vi "Main UI.vi"(8 "error in (no error)":errorcluster, 11 "picoG in":refnum<class "picoG.lvclass">) -> (0 "error out":errorcluster, 3 "picoG out":refnum<class "picoG.lvclass">)   [LabVIEW 2020, in "PicoG-App.lvlib" / "picoG.lvclass"]
uses:
  picoG.lvclass
  UI State.ctl
  picoG.lvclass/picoG.ctl
  AppListPanel/AppListPanel.lvclass
  C:/Program Files (x86)/National Instruments/LabVIEW 2020/vi.lib/IlluminatedG/IG OOPanel/OOPanel/Panel/Panel.lvclass
  DeviceListPanel/DeviceListPanel.lvclass
  GettingStarted/GettingStarted.lvclass
  PlatformListPanel/PlatformListPanel.lvclass
  AppDetailPanel/AppDetailPanel.lvclass
  DeviceDetailPanel/DeviceDetailPanel.lvclass
  PlatformConfigPanel/PlatformConfigPanel.lvclass
  AppListPanel/Panel.vi
  ViaApp/ViaApp.lvclass
  Builds/picoG/ppl/PicoG-Core.lvlibp/PicoG-Processor/PicoG-Core/Platform/Platform.lvclass
  Device/Device.lvclass
  <vilib>/IlluminatedG/IG OOPanel/OOPanel/Manager/Manager.lvclass
  PicoG-App.lvlib
  App Watcher/App Watcher.lvclass
panel:
  in  "System":bool
  in  "Devices":bool
  in  "Apps":bool
  in  "Platforms":bool
  in  "OK Button":bool
  out "StatusLeft":string
  out "StatusLeft 2":string
  out "StatusRight 2":string
  out "ProgressBar":dbl(slide) scale=0.0..100.0
  out "StatusRight":string
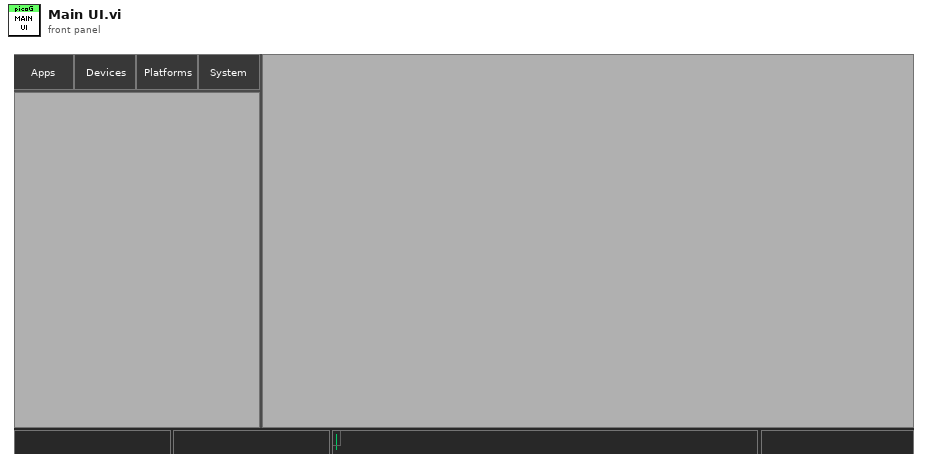
[diagram p1: front panel]
types:
  T1 = typedef "PicoG-App.lvlib/picoG.lvclass/UI State.ctl" = enum16{"Init", "Run", "Close"}
  T2 = enum32{"Invalid", "Standard", "Closed", "Hidden", "Minimized", "Maximized"}
  T3 = typedef "PicoG-App.lvlib/picoG.lvclass/Inbound Events.ctl" = cluster{"Add App":refnum<user-event>, "App Update":refnum<user-event>, "Select App":refnum<user-event>, "Select Platform":refnum<user-event>, "Add Device":refnum<user-event>, "Select Device":refnum<user-event>, "Remove App":refnum<user-event>, "Deploy Event":refnum<user-event>, "Remove Device":refnum<user-event>, "Refresh Device":refnum<user-event>}
  T4 = typedef "PicoG-App.lvlib/Device.lvclass/Device Key.ctl" = cluster{"Platform":string, "Board":string, "ID":string}
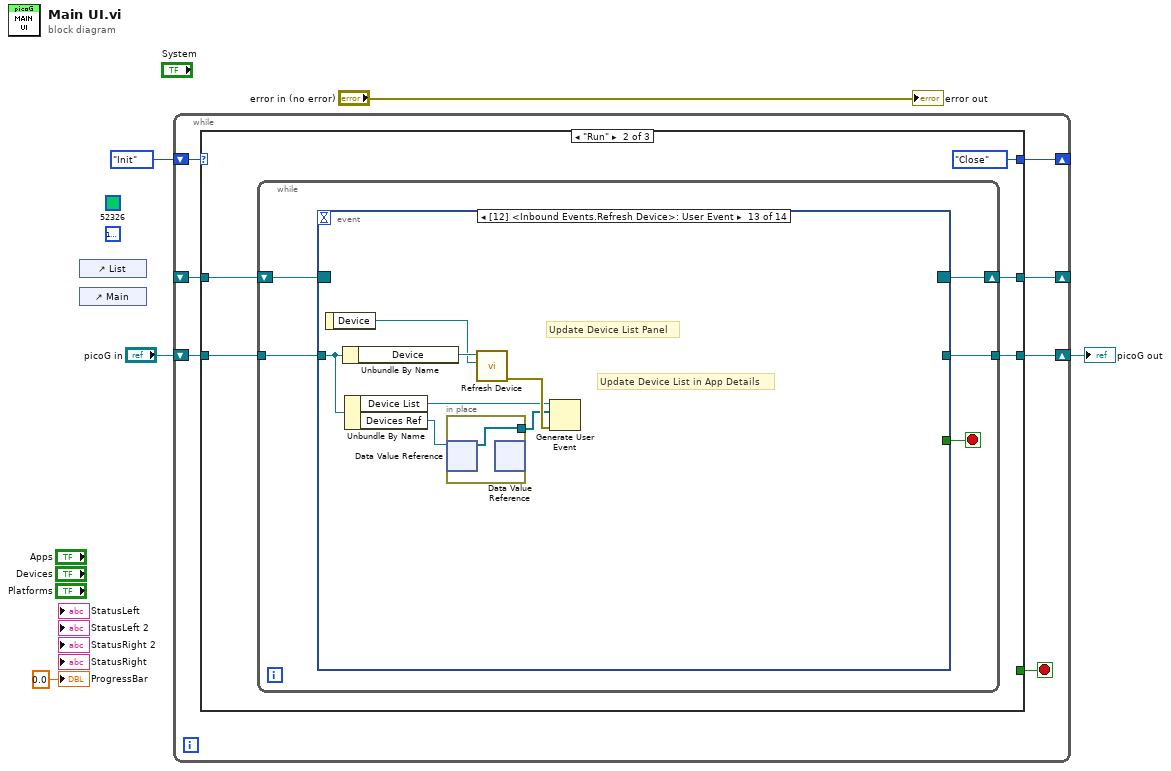
[diagram p0: block diagram]
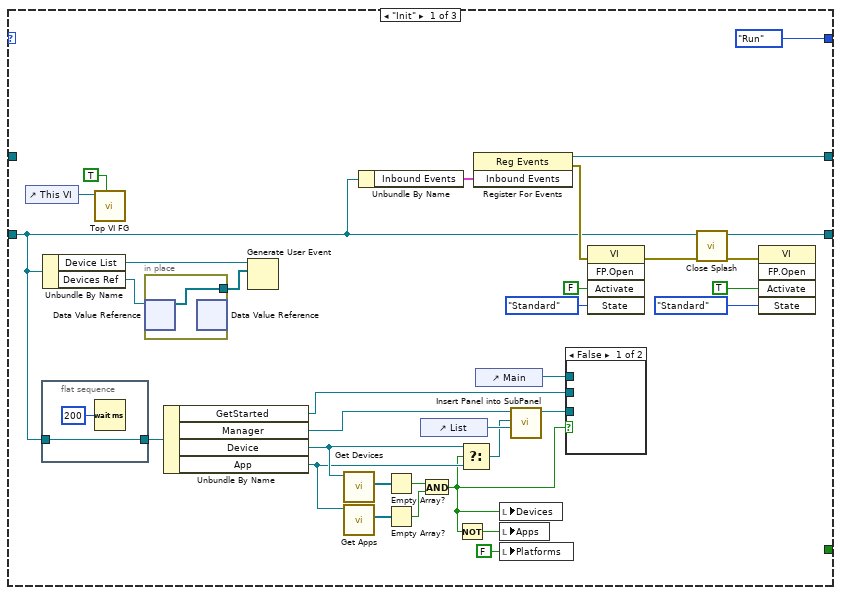
[diagram p2: hidden frame]
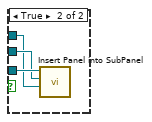
[diagram p3: hidden frame]
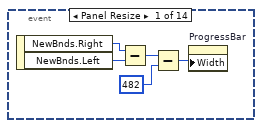
[diagram p4: hidden frame]
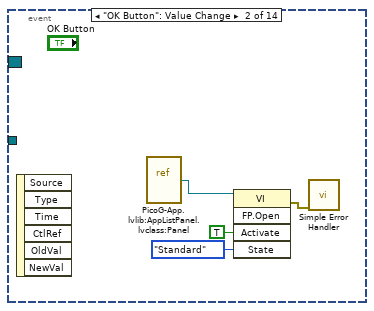
[diagram p5: hidden frame]
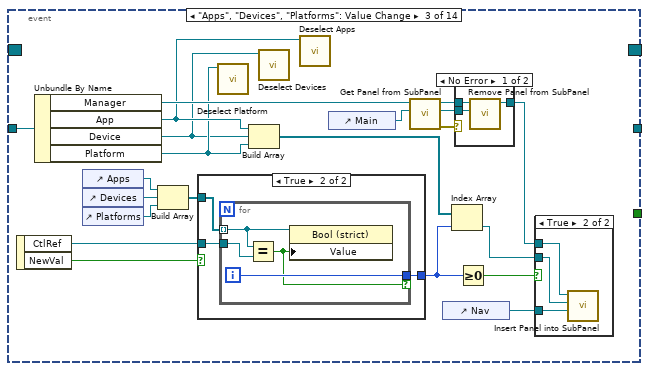
[diagram p6: hidden frame]
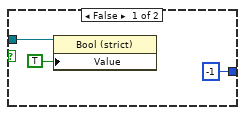
[diagram p9: hidden frame]
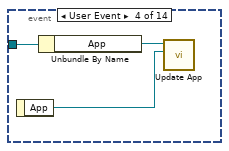
[diagram p10: hidden frame]
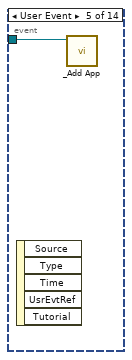
[diagram p11: hidden frame]
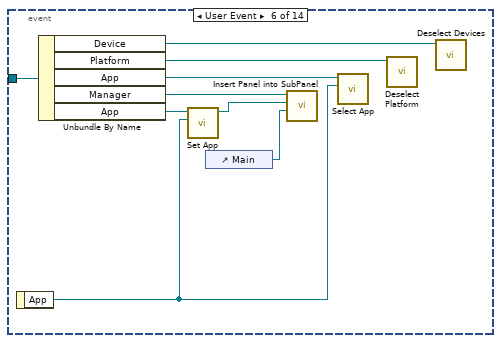
[diagram p12: hidden frame]
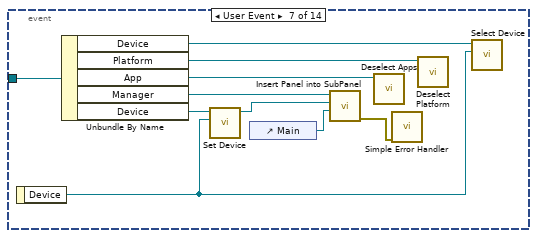
[diagram p13: hidden frame]
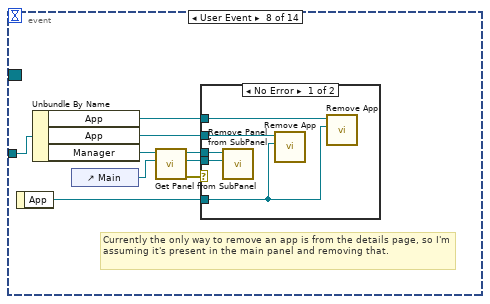
[diagram p14: hidden frame]
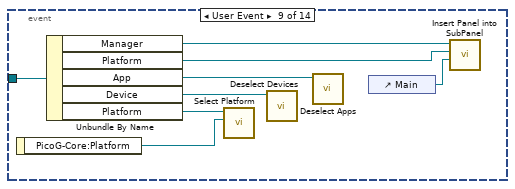
[diagram p16: hidden frame]
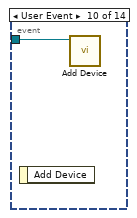
[diagram p17: hidden frame]
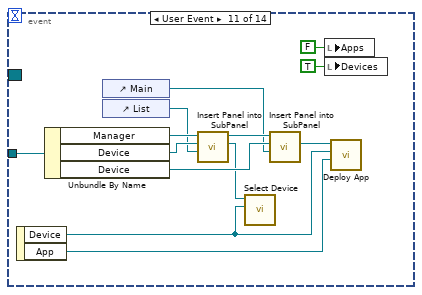
[diagram p18: hidden frame]
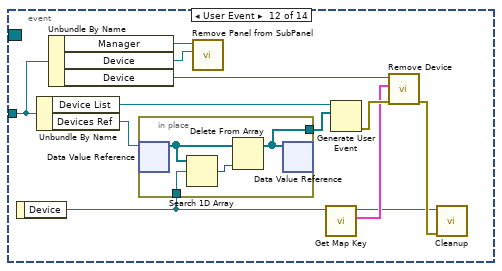
[diagram p19: hidden frame]
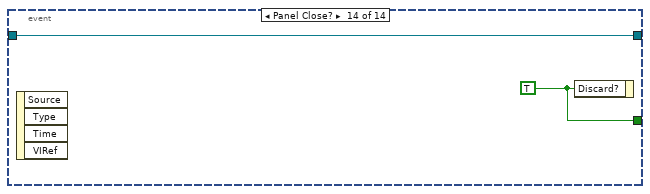
[diagram p20: hidden frame]
diagram:
  (unwired) u32 16777216
  (unwired) u32 52326
  n1 = control-ref of="List"() -> ()  [unwired: 1 out]
  n2 = control-ref of="Main"() -> ()  [unwired: 1 out]
  n3 = while {
    shift-right: [w11] -> _
    shift-left: UI_State."Init" ("UI State") -> [w12]
    shift-right: [w8] -> w2
    shift-left: "picoG in" -> [w9]
    shift-right: [w7] -> _
    shift-left: _ -> [w6]
    stop <- w10 stop-if-true
    n4 = case shown="\"Run\"" w12 {
      selector: w12 -> [_ _ w200]
      tunnel: [UI_State."Run" ("UI State") UI_State."Close" ("UI State") w200] -> w11
      tunnel: [_ _ TRUE] -> w10
      tunnel: w9 -> [w13 w55 w196]
      tunnel: [w37 w54 w195] -> w8
      tunnel: [w34 w52 _] -> w7
      tunnel: w6 -> [_ w53 w197]
      frame "Init" {
        n5 = control-ref of="This VI"() -> (w33:refnum<vi>)
        n6 = flat-sequence {
          tunnel: w13 -> [w48]
          tunnel: [w48] -> w17
          frame #0 {
            n7 = Wait (ms)(milliseconds to wait=u32 200) -> ()  [unwired: 1 out]
          }
        }
        n8 = Unbundle By Name(w13) -> ("Device List"=w15:refnum<user-event>, "Devices Ref"=w16:refnum<data-value>)
        n9 = call "Top VI FG.vi"("Set (F)"=TRUE, "Top-Level VI In"=w33) -> ()  [unwired: 8 in, 2 out]
        n10 = in-place {
          in-place-border: [w46] -> w14
          n11 = in-place-dvr #1(w16) -> (w46:refnum<class "Device.lvclass">[])  [unwired: 1 out]
          n12 = in-place-dvr #1() -> ()  [unwired: 1 in, 2 out]
        }
        n13 = Unbundle By Name(w17) -> ("GetStarted"=w20:refnum<class "GettingStarted.lvclass">, "Manager"=w23:refnum<class "Manager.lvclass">, "Device"=w26:refnum<class "DeviceListPanel.lvclass">, "App"=w25:refnum<class "AppListPanel.lvclass">)
        n14 = Generate User Event(user event=w15, event data cluster=w14) -> ()  [unwired: 2 in, 2 out]
        n15 = call "Get Devices.vi"("DeviceListPanel in"=w26) -> ("Devices"=w29:refnum<class "Device.lvclass">[])  [unwired: 8 in, 2 out]
        n16 = call "Get Apps.vi"("AppListPanel in"=w25) -> ("Apps"=w30:refnum<class "ViaApp.lvclass">[])  [unwired: 8 in, 2 out]
        n17 = Unbundle By Name(w13) -> ("Inbound Events"=w35:T3)
        n18 = Empty Array?(array=w29) -> (empty?=w27:bool)
        n19 = Empty Array?(array=w30) -> (empty?=w28:bool)
        n20 = control-ref of="List"() -> (w36:refnum<vi>)
        n21 = And(x=w27, y=w28) -> (x .and. y?=w18:bool)
        n22 = Not(x=w18) -> (.not. x?=w19:bool)
        n23 = Select(t=w26, s=w18, f=w25) -> (s? t:f=w24:refnum<class "Panel.lvclass">)
        n24 = register-events(w35) -> (reference out=w34:refnum<event-registration>, error out=w45:errorcluster)  [unwired: 2 in]
        n25 = control-ref of="Main"() -> (w22:refnum<vi>)
        n26 = local write "Devices"(w18) -> ()
        n27 = local write "Apps"(w19) -> ()
        n28 = local write "Platforms"(FALSE ("Nav Devices")) -> ()
        n29 = call <vilib>:"Insert Panel into SubPanel.vi"("SubPanel"=w36, "Panel In"=w24, "Manager in"=w23) -> ("Manager out"=w21:refnum<class "Manager.lvclass">)  [unwired: 6 in, 2 out]
        n30 = case shown="False" w18 {
          tunnel: w22 -> [_ w49]
          tunnel: w21 -> [_ w51]
          tunnel: w20 -> [_ w50]
          frame False {
          }
          frame True {
            n31 = call <vilib>:"Insert Panel into SubPanel.vi"("SubPanel"=w49, "Panel In"=w50, "Manager in"=w51) -> ()  [unwired: 6 in, 3 out]
          }
        }
        n32 = invoke class="VI" method="FP.Open"(error in=w45, "Activate"=FALSE ("Activate?"), "State"=T2."Standard") -> (error out=w41:errorcluster)  [unwired: 2 in, 4 out]
        n33 = call "Close Splash.vi"("error in (no error)"=w41, "picoG in"=w13) -> ("error out"=w40:errorcluster, "picoG out"=w37:refnum<class "picoG.lvclass">)  [unwired: 8 in]
        n34 = invoke class="VI" method="FP.Open"(error in=w40, "Activate"=TRUE ("Activate?"), "State"=T2."Standard") -> ()  [unwired: 2 in, 5 out]
      }
      frame "Run" {
        n35 = while {
          tunnel: w55 -> [w60]
          tunnel: [w59] -> w54
          shift-right: [w57] -> w52
          shift-left: w53 -> [w58]
          stop <- w61 stop-if-true
          n36 = event shown="[12] <Inbound Events.Refresh Device>: User Event" {
            selector: w58 -> [_ _ _ _ _ _ _ _ _ _ _ _ _ _]
            dyn-events: [_ _ _ _ _ _ _ _ _ _ _ _ _ _] -> w57
            timeout: _ -> [_ _ _ _ _ _ _ _ _ _ _ _ _ _]
            tunnel: [_ _ _ _ _ _ _ _ _ _ _ _ _ w193] -> w61
            tunnel: w60 -> [_ _ w82 w111 w112 w121 w129 w140 w153 w154 w167 w176 w187 w192]
            tunnel: [_ _ _ _ _ _ _ _ _ _ _ _ _ w192] -> w59
            event Panel Resize {
              n37 = event-data() -> ("NewBnds.Right"=w65:i16, "NewBnds.Left"=w66:i16)  [unwired: 1 in]
              n38 = Subtract(x=w65, y=w66) -> (x-y=w64:i16)
              n39 = Subtract(x=w64, y=i16 482) -> (x-y=w62:i16)
              n40 = property on="ProgressBar" class="Slide (strict)"("Width"=w62) -> ()  [unwired: 2 in, 2 out]
            }
            event "OK Button": Value Change {
              n41 = event-data() -> ()  [unwired: 1 in, 6 out]
              n42 = vi-ref "PicoG-App.lvlib:AppListPanel.lvclass:Panel.vi"() -> (w70:refnum<vi>)
              n43 = invoke class="VI" method="FP.Open"(reference=w70, "Activate"=TRUE ("Activate?"), "State"=T2."Standard") -> (error out=w67:errorcluster)  [unwired: 2 in, 4 out]
              n44 = call <vilib>:"Simple Error Handler.vi"("error in (no error)"=w67) -> ()  [unwired: 4 in, 5 out]
            }
            event "Apps", "Devices", "Platforms": Value Change {
              n45 = event-data() -> ("CtlRef"=w90:refnum<vi>, "NewVal"=w91:bool)  [unwired: 1 in]
              n46 = Unbundle By Name(w82) -> ("Manager"=w79:refnum<class "Manager.lvclass">, "App"=w74:refnum<class "AppListPanel.lvclass">, "Device"=w71:refnum<class "DeviceListPanel.lvclass">, "Platform"=w73:refnum<class "PlatformListPanel.lvclass">)
              n47 = control-ref of="Apps"() -> (w88:refnum<vi>)
              n48 = control-ref of="Devices"() -> (w89:refnum<vi>)
              n49 = control-ref of="Platforms"() -> (w87:refnum<vi>)
              n50 = Build Array(w88, w89, w87) -> (w80:refnum<vi>[])
              n51 = case shown="True" w91 {
                tunnel: w90 -> [w101 w104]
                tunnel: w80 -> [_ w103]
                tunnel: [-1 w102] -> w86
                frame False {
                  n52 = property class="Bool (strict)"(reference=w101, "Value"=TRUE) -> ()  [unwired: 1 in, 2 out]
                }
                frame True {
                  n53 = for {
                    tunnel: w104 -> [w108]
                    tunnel: w103 -> [w107] mode=indexing
                    tunnel: [w106] -> w102 if=w105
                    i -> [w106]
                    n54 = Equal?(x=w107, y=w108) -> (x = y?=w105:bool)
                    n55 = property class="Bool (strict)"(reference=w107, "Value"=w105) -> ()  [unwired: 1 in, 2 out]
                  }
                }
              }
              n56 = call "Deselect Platform.vi"("PlatformListPanel in"=w73) -> ()  [unwired: 9 in, 2 out]
              n57 = Build Array(w74, w71, w73) -> (w81:refnum<class "Panel.lvclass">[])
              n58 = call "Deselect Devices.vi"("DeviceListPanel in"=w71) -> ()  [unwired: 9 in, 2 out]
              n59 = call "Deselect Apps.vi"("AppListPanel in"=w74) -> ()  [unwired: 9 in, 2 out]
              n60 = control-ref of="Main"() -> (w78:refnum<vi>)
              n61 = call <vilib>:"Get Panel from SubPanel.vi"("SubPanel"=w78, "Manager in"=w79) -> ("error out"=w72:errorcluster, "Panel"=w76:refnum<class "Panel.lvclass">, "Manager out"=w77:refnum<class "Manager.lvclass">)  [unwired: 7 in]
              n62 = control-ref of="Nav"() -> (w84:refnum<vi>)
              n63 = Index Array(array=w81, index=w86) -> (element=w83:refnum<class "Panel.lvclass">)
              n64 = case shown="No Error" w72 {
                tunnel: w77 -> [w94 w95]
                tunnel: w76 -> [w93 _]
                tunnel: [w92 w95] -> w75
                frame No Error {
                  n65 = call <vilib>:"Remove Panel from SubPanel.vi"("Panel In"=w93, "Manager in"=w94) -> ("Manager out"=w92:refnum<class "Manager.lvclass">)  [unwired: 7 in, 2 out]
                }
                frame Error {
                }
              }
              n66 = Greater Or Equal To 0?(x=w86) -> (x >= 0?=w85:bool)
              n67 = case shown="True" w85 {
                tunnel: w84 -> [_ w98]
                tunnel: w83 -> [_ w97]
                tunnel: w75 -> [_ w96]
                frame False {
                }
                frame True {
                  n68 = call <vilib>:"Insert Panel into SubPanel.vi"("SubPanel"=w98, "Panel In"=w97, "Manager in"=w96) -> ()  [unwired: 6 in, 3 out]
                }
              }
            }
            event User Event {
              n69 = event-data() -> ("App"=w109:refnum<class "ViaApp.lvclass">)  [unwired: 1 in]
              n70 = Unbundle By Name(w111) -> ("App"=w110:refnum<class "AppListPanel.lvclass">)
              n71 = call "Update App.vi"("ViaApp"=w109, "AppListPanel in"=w110) -> ()  [unwired: 8 in, 2 out]
            }
            event User Event {
              n72 = event-data() -> ()  [unwired: 1 in, 5 out]
              n73 = call "_Add App.vi"("picoG in"=w112) -> ()  [unwired: 9 in, 2 out]
            }
            event User Event {
              n74 = event-data() -> ("App"=w117:refnum<class "ViaApp.lvclass">)  [unwired: 1 in]
              n75 = Unbundle By Name(w121) -> ("Device"=w113:refnum<class "DeviceListPanel.lvclass">, "Platform"=w119:refnum<class "PlatformListPanel.lvclass">, "App"=w120:refnum<class "AppListPanel.lvclass">, "Manager"=w116:refnum<class "Manager.lvclass">, "App"=w118:refnum<class "AppDetailPanel.lvclass">)
              n76 = call "Set App.vi"("App"=w117, "AppDetailPanel in"=w118) -> ("AppDetailPanel out"=w114:refnum<class "AppDetailPanel.lvclass">)  [unwired: 8 in, 1 out]
              n77 = control-ref of="Main"() -> (w115:refnum<vi>)
              n78 = call <vilib>:"Insert Panel into SubPanel.vi"("SubPanel"=w115, "Panel In"=w114, "Manager in"=w116) -> ()  [unwired: 6 in, 3 out]
              n79 = call "Select App.vi"("App"=w117, "AppListPanel in"=w120) -> ()  [unwired: 8 in, 2 out]
              n80 = call "Deselect Platform.vi"("PlatformListPanel in"=w119) -> ()  [unwired: 9 in, 2 out]
              n81 = call "Deselect Devices.vi"("DeviceListPanel in"=w113) -> ()  [unwired: 9 in, 2 out]
            }
            event User Event {
              n82 = event-data() -> ("Device"=w125:refnum<class "Device.lvclass">)  [unwired: 1 in]
              n83 = Unbundle By Name(w129) -> ("Device"=w128:refnum<class "DeviceListPanel.lvclass">, "Platform"=w131:refnum<class "PlatformListPanel.lvclass">, "App"=w124:refnum<class "AppListPanel.lvclass">, "Manager"=w130:refnum<class "Manager.lvclass">, "Device"=w127:refnum<class "DeviceDetailPanel.lvclass">)
              n84 = call "Set Device.vi"("Device"=w125, "DeviceDetailPanel in"=w127) -> ("DeviceDetailPanel out"=w126:refnum<class "DeviceDetailPanel.lvclass">)  [unwired: 8 in, 1 out]
              n85 = control-ref of="Main"() -> (w122:refnum<vi>)
              n86 = call <vilib>:"Insert Panel into SubPanel.vi"("SubPanel"=w122, "Panel In"=w126, "Manager in"=w130) -> ("error out"=w123:errorcluster)  [unwired: 6 in, 2 out]
              n87 = call "Deselect Apps.vi"("AppListPanel in"=w124) -> ()  [unwired: 9 in, 2 out]
              n88 = call <vilib>:"Simple Error Handler.vi"("error in (no error)"=w123) -> ()  [unwired: 4 in, 5 out]
              n89 = call "Deselect Platform.vi"("PlatformListPanel in"=w131) -> ()  [unwired: 9 in, 2 out]
              n90 = call "Select Device.vi"("Device"=w125, "DeviceListPanel in"=w128) -> ()  [unwired: 8 in, 2 out]
            }
            event User Event {
              # "Currently the only way to remove an app is from the details page, so I'm assuming it's present in the main panel and removing that."
              n91 = event-data() -> ("App"=w135:refnum<class "ViaApp.lvclass">)  [unwired: 1 in]
              n92 = Unbundle By Name(w140) -> ("App"=w132:refnum<class "App Watcher.lvclass">, "App"=w133:refnum<class "AppListPanel.lvclass">, "Manager"=w139:refnum<class "Manager.lvclass">)
              n93 = control-ref of="Main"() -> (w138:refnum<vi>)
              n94 = call <vilib>:"Get Panel from SubPanel.vi"("SubPanel"=w138, "Manager in"=w139) -> ("error out"=w136:errorcluster, "Panel"=w137:refnum<class "Panel.lvclass">, "Manager out"=w134:refnum<class "Manager.lvclass">)  [unwired: 7 in]
              n95 = case shown="No Error" w136 {
                tunnel: w137 -> [w145 _]
                tunnel: w135 -> [w141 _]
                tunnel: w134 -> [w144 _]
                tunnel: w133 -> [w143 _]
                tunnel: w132 -> [w142 _]
                frame No Error {
                  n96 = call <vilib>:"Remove Panel from SubPanel.vi"("Panel In"=w145, "Manager in"=w144) -> ()  [unwired: 7 in, 3 out]
                  n97 = call "Remove App.vi"("App"=w141, "AppListPanel in"=w143) -> ()  [unwired: 8 in, 2 out]
                  n98 = call "Remove App.vi"("App"=w141, "App Watcher in"=w142) -> ()  [unwired: 8 in, 2 out]
                }
                frame Error {
                  # "#ERROR?"
                }
              }
            }
            event User Event {
              n99 = event-data() -> ("PicoG-Core:Platform"=w151:refnum<class "Platform.lvclass">)  [unwired: 1 in]
              n100 = Unbundle By Name(w153) -> ("Manager"=w148:refnum<class "Manager.lvclass">, "Platform"=w147:refnum<class "PlatformConfigPanel.lvclass">, "App"=w150:refnum<class "AppListPanel.lvclass">, "Device"=w146:refnum<class "DeviceListPanel.lvclass">, "Platform"=w152:refnum<class "PlatformListPanel.lvclass">)
              n101 = call "Select Platform.vi"("Platform"=w151, "PlatformListPanel in"=w152) -> ()  [unwired: 8 in, 2 out]
              n102 = call "Deselect Devices.vi"("DeviceListPanel in"=w146) -> ()  [unwired: 9 in, 2 out]
              n103 = call "Deselect Apps.vi"("AppListPanel in"=w150) -> ()  [unwired: 9 in, 2 out]
              n104 = control-ref of="Main"() -> (w149:refnum<vi>)
              n105 = call <vilib>:"Insert Panel into SubPanel.vi"("SubPanel"=w149, "Panel In"=w147, "Manager in"=w148) -> ()  [unwired: 6 in, 3 out]
            }
            event User Event {
              n106 = event-data() -> ()  [unwired: 1 in, 1 out]
              n107 = call "Add Device.vi"("picoG in"=w154) -> ()  [unwired: 9 in, 2 out]
            }
            event User Event {
              n108 = event-data() -> ("Device"=w158:refnum<class "Device.lvclass">, "App"=w157:refnum<class "ViaApp.lvclass">)  [unwired: 1 in]
              n109 = Unbundle By Name(w167) -> ("Manager"=w166:refnum<class "Manager.lvclass">, "Device"=w165:refnum<class "DeviceListPanel.lvclass">, "Device"=w163:refnum<class "DeviceDetailPanel.lvclass">)
              n110 = control-ref of="Main"() -> (w155:refnum<vi>)
              n111 = control-ref of="List"() -> (w156:refnum<vi>)
              n112 = call <vilib>:"Insert Panel into SubPanel.vi"("SubPanel"=w156, "Panel In"=w165, "Manager in"=w166) -> ("Panel"=w160:refnum<class "DeviceListPanel.lvclass">, "Manager out"=w164:refnum<class "Manager.lvclass">)  [unwired: 6 in, 1 out]
              n113 = call "Select Device.vi"("Device"=w158, "DeviceListPanel in"=w160) -> ()  [unwired: 8 in, 2 out]
              n114 = call <vilib>:"Insert Panel into SubPanel.vi"("SubPanel"=w155, "Panel In"=w163, "Manager in"=w164) -> ("Panel"=w159:refnum<class "DeviceDetailPanel.lvclass">)  [unwired: 6 in, 2 out]
              n115 = local write "Apps"(FALSE ("Apps")) -> ()
              n116 = local write "Devices"(TRUE ("Devices")) -> ()
              n117 = call "Deploy App.vi"("App"=w157, "Device"=w158, "DeviceDetailPanel in"=w159) -> ()  [unwired: 7 in, 2 out]
            }
            event User Event {
              n118 = event-data() -> ("Device"=w170:refnum<class "Device.lvclass">)  [unwired: 1 in]
              n119 = Unbundle By Name(w176) -> ("Device List"=w178:refnum<user-event>, "Devices Ref"=w179:refnum<data-value>)
              n120 = Unbundle By Name(w176) -> ("Manager"=w172:refnum<class "Manager.lvclass">, "Device"=w171:refnum<class "DeviceDetailPanel.lvclass">, "Device"=w175:refnum<class "DeviceListPanel.lvclass">)
              n121 = in-place {
                in-place-border: w170 -> [w183]
                in-place-border: [w180] -> w177
                n122 = in-place-dvr #2(w179) -> (w182:refnum<class "Device.lvclass">[])  [unwired: 1 out]
                n123 = Search 1D Array(1D array=w182, element=w183) -> (index of element=w181:i32)  [unwired: 1 in]
                n124 = Delete From Array(array=w182, index=w181) -> (array with subset deleted=w180:refnum<class "Device.lvclass">[])  [unwired: 1 in, 1 out]
                n125 = in-place-dvr #2(w180) -> ()  [unwired: 2 out]
              }
              n126 = call <vilib>:"Remove Panel from SubPanel.vi"("Panel In"=w171, "Manager in"=w172) -> ()  [unwired: 7 in, 3 out]
              n127 = call "Get Map Key.vi"("Device in"=w170) -> ("Key"=w169:T4, "Device out"=w168:refnum<class "Device.lvclass">)  [unwired: 8 in, 1 out]
              n128 = Generate User Event(user event=w178, event data cluster=w177) -> (error out=w174:errorcluster)  [unwired: 2 in, 1 out]
              n129 = call "Remove Device.vi"("error in (no error)"=w174, "Key"=w169, "DeviceListPanel in"=w175) -> ("error out"=w173:errorcluster)  [unwired: 7 in, 1 out]
              n130 = call "Cleanup.vi"("error in (no error)"=w173, "Device in"=w168) -> ()  [unwired: 9 in, 1 out]
            }
            event User Event {
              # "Update Device List in App Details"
              # "Update Device List Panel"
              n131 = event-data() -> ("Device"=w188:refnum<class "Device.lvclass">)  [unwired: 1 in]
              n132 = Unbundle By Name(w187) -> ("Device"=w189:refnum<class "DeviceListPanel.lvclass">)
              n133 = Unbundle By Name(w187) -> ("Device List"=w184:refnum<user-event>, "Devices Ref"=w186:refnum<data-value>)
              n134 = in-place {
                in-place-border: [w191] -> w185
                n135 = in-place-dvr #3(w186) -> (w191:refnum<class "Device.lvclass">[])  [unwired: 1 out]
                n136 = in-place-dvr #3() -> ()  [unwired: 1 in, 2 out]
              }
              n137 = call "Refresh Device.vi"("Device"=w188, "DeviceListPanel in"=w189) -> ("error out"=w190:errorcluster)  [unwired: 8 in, 1 out]
              n138 = Generate User Event(user event=w184, event data cluster=w185, error in=w190) -> ()  [unwired: 1 in, 2 out]
            }
            event Panel Close? {
              w193 = TRUE ("Discard?")
              n139 = event-data() -> ()  [unwired: 1 in, 4 out]
              n140 = event-data("Discard?"=w193) -> ()  [unwired: 1 in, 1 out]
            }
          }
        }
      }
      frame "Close" {
        # "Save configs here before everything gets cleaned up in... Cleanup.vi"
        n141 = Unregister For Events(event registration refnum=w197) -> ()  [unwired: 1 in, 1 out]
        n142 = call "Save Config.vi"("picoG in"=w196) -> ("error out"=w194:errorcluster, "picoG out"=w195:refnum<class "picoG.lvclass">)  [unwired: 9 in]
        n143 = call <vilib>:"Simple Error Handler.vi"("error in (no error)"=w194) -> ()  [unwired: 4 in, 5 out]
        n144 = control-ref of="This VI"() -> (w198:refnum<vi>)
        n145 = invoke class="VI" method="FP.Close"(reference=w198) -> ()  [unwired: 2 in, 3 out]
      }
    }
  }
  "picoG out" <- w2
  "error out" <- "error in (no error)"
  "ProgressBar" <- 0.0 ("ProgressBar")
